vi "Set Address.vi"(10 "Column":i32, 11 "Row":i32) -> (3 "2D Array Index":refnum<class "Address.lvclass">)   [LabVIEW 2019, in "Address.lvclass"]
uses:
  Address.lvclass
  Address.lvclass/Address.ctl
  Write Row.vi
  Write Column.vi
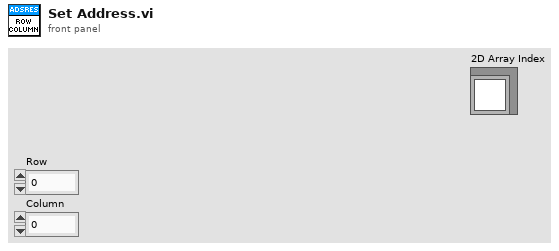
[diagram p1: front panel]
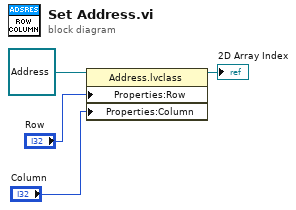
[diagram p0: block diagram]
diagram:
  n1 = property class="Address.lvclass"(reference=refnum<class "Address.lvclass"> refnum ("2D Array.lvclass"), "Properties:Row"="Row", "Properties:Column"="Column") -> (reference out=→"2D Array Index":refnum<class "Address.lvclass">)  [unwired: 1 in, 1 out]
